vi "Configure NF Correction.vi"(0 "VISA resource name":refnum<visa-resource-name>, 1 "Correction Before DUT Temperature (0 K)":dbl format="%^#_6g", 7 "User Tcold Value (296.5 K)":dbl=296.5 format="%^#_6g", 9 "Correction After DUT Temperature (0 K)":dbl format="%^#_6g", 11 "error in (no error)":errorcluster, 12 "User Tcold Control (Disabled)":bool) -> (4 "VISA resource name out":refnum<visa-resource-name>, 15 "error out":errorcluster)   [LabVIEW 2014, in "Agilent ESA PSA Series.lvlib"]
doc: "Configures the correction options for the Noise Figure personality.\n\n<B>Note:</B> \n\nThis VI is only valid in Noise Figure personality. Use <B>Switch Personality</B> VI to switch to Noise Figure before calling this VI."
uses:
  Agilent ESA PSA Series.lvlib
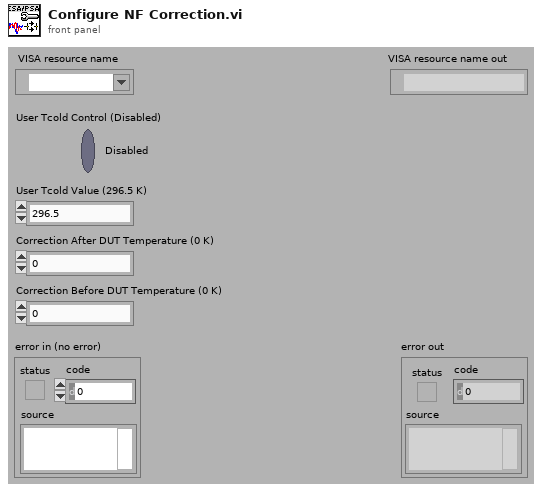
[diagram p1: front panel]
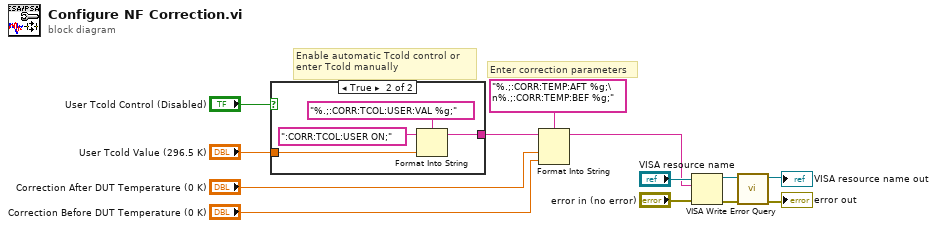
[diagram p0: block diagram]
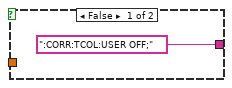
[diagram p2: hidden frame]
diagram:
  # "Enter correction parameters"
  # "Enable automatic Tcold control or\nenter Tcold manually"
  n1 = case shown="True" "User Tcold Control (Disabled)" {
    tunnel: "User Tcold Value (296.5 K)" -> [_ w18]
    tunnel: [":CORR:TCOL:USER OFF;" w15] -> w5
    frame False {
    }
    frame True {
      n2 = Format Into String(format string="%.;:CORR:TCOL:USER:VAL %g;", initial string=":CORR:TCOL:USER ON;", w18) -> (resulting string=w15:string)  [unwired: 1 in, 1 out]
    }
  }
  n3 = Format Into String(format string="%.;:CORR:TEMP:AFT %g;\n%.;:CORR:TEMP:BEF %g;", initial string=w5, "Correction After DUT Temperature (0 K)", "Correction Before DUT Temperature (0 K)") -> (resulting string=w1:string)  [unwired: 1 in, 1 out]
  n4 = VISA Write(VISA resource name="VISA resource name", write buffer=w1, error in (no error)="error in (no error)") -> (VISA resource name out=w11:refnum<visa-resource-name>, error out=w10:errorcluster)  [unwired: 1 out]
  n5 = call "Error Query.vi"("error in (no error)"=w10, "VISA resource name"=w11) -> ("error out"=→"error out":errorcluster, "VISA resource name out"=→"VISA resource name out":refnum<visa-resource-name>)  [unwired: 6 in, 2 out]
